vi "GetStatus.vi"(8 "error in (no error)":errorcluster, 11 "MotorController in":refnum<class "MotorController.lvclass">) -> (0 "error out":errorcluster, 2 "Ready":bool, 3 "MotorController out":refnum<class "MotorController.lvclass">)   [LabVIEW 2019, in "MotorController.lvclass"]
uses:
  MotorController.lvclass
  MotorController.lvclass/MotorController.ctl
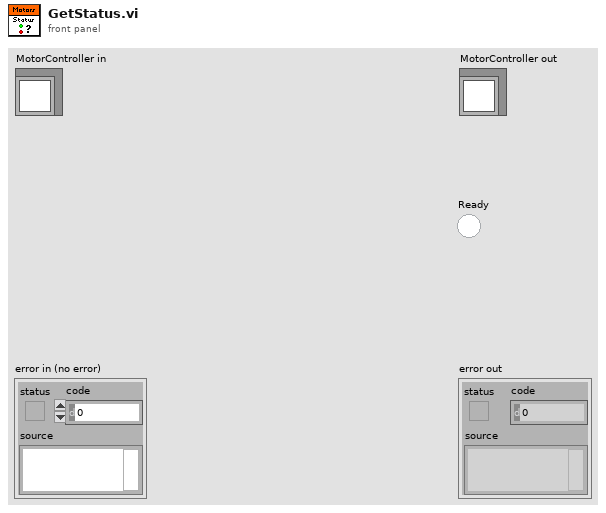
[diagram p1: front panel]
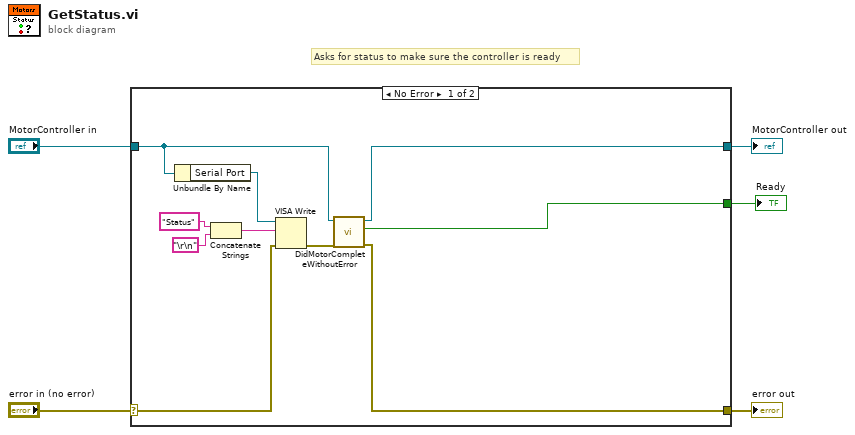
[diagram p0: block diagram]
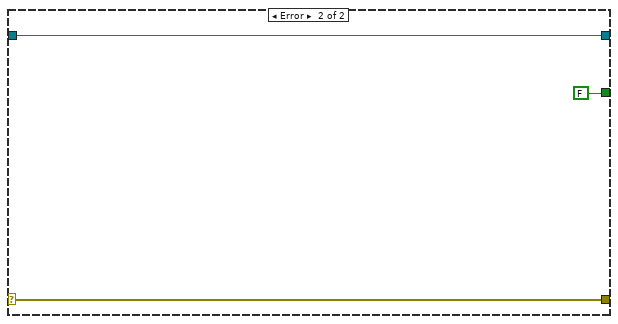
[diagram p2: hidden frame]
diagram:
  # "Asks for status to make sure the controller is ready"
  n1 = case shown="No Error" "error in (no error)" {
    selector: "error in (no error)" -> [w14 w18]
    tunnel: [w6 w18] -> w4
    tunnel: [w8 w17] -> w2
    tunnel: "MotorController in" -> [w9 w17]
    tunnel: [w7 FALSE] -> w1
    frame No Error {
      n2 = Unbundle By Name(w9) -> ("Serial Port"=w15:refnum<visa-resource-name>)
      n3 = Concatenate Strings("Status", "\r\n") -> (w11:string)
      n4 = VISA Write(VISA resource name=w15, write buffer=w11, error in (no error)=w14) -> (error out=w10:errorcluster)  [unwired: 2 out]
      n5 = call "DidMotorCompleteWithoutError.vi"("error in (no error)"=w10, "MotorController in"=w9) -> ("error out"=w6:errorcluster, "Completed Sucessfully"=w7:bool, "MotorController out"=w8:refnum<class "MotorController.lvclass">)  [unwired: 7 in]
    }
    frame Error {
    }
  }
  "error out" <- w4
  "MotorController out" <- w2
  "Ready" <- w1
